vi "Piechart_.vi"(9 "Pie Chart Size (200 pixels)":dbl=200.0, 10 "Division Colors":u32[](array[colorbox]), 11 "Pie Chart Data (arb unit)":dbl[](array[numeric])) -> (3 "Pie Chart":picture)   [LabVIEW 2014]
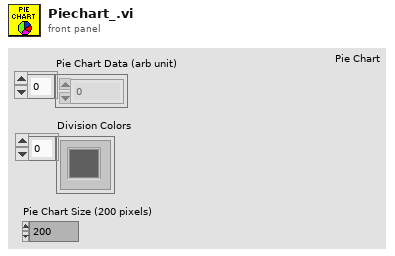
[diagram p1: front panel]
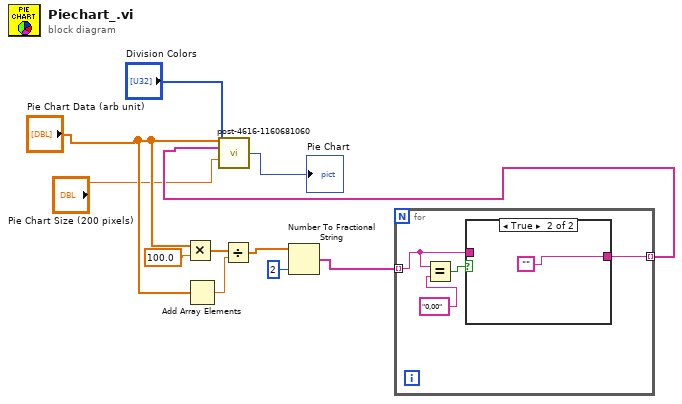
[diagram p0: block diagram]
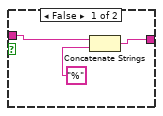
[diagram p2: hidden frame]
diagram:
  n1 = Multiply(x="Pie Chart Data (arb unit)", y=100.0) -> (x*y=w9:dbl[])
  n2 = Add Array Elements(numeric array="Pie Chart Data (arb unit)") -> (sum=w8:dbl)
  n3 = Divide(x=w9, y=w8) -> (x/y=w7:dbl[])
  n4 = Number To Fractional String(number=w7, precision (6)=i16 2) -> (F-format string=w5:string[])  [unwired: 2 in]
  n5 = for {
    tunnel: w5 -> [w14] mode=indexing
    tunnel: [w15] -> w4 mode=indexing
    n6 = Equal?(x=w14, y="0,00" ("search string/char (-)")) -> (x = y?=w12:bool)
    n7 = case shown="True" w12 {
      tunnel: w14 -> [w17 _]
      tunnel: [w16 ""] -> w15
      frame False {
        n8 = Concatenate Strings(w17, "%" ("string")) -> (w16:string)
      }
      frame True {
      }
    }
  }
  n9 = call "post-4616-1160681060.vi"("Pie Chart Data (arb unit)"="Pie Chart Data (arb unit)", "Label Text (No Labels)"=w4, "Division Colors"="Division Colors", "Pie Chart Size (200 pixels)"="Pie Chart Size (200 pixels)") -> ("Pie Chart"=→"Pie Chart":picture)  [unwired: 11 in]
